vi "Show table.vi"() -> ()   [LabVIEW 2015]
uses:
  <vilib>/addons/database/_DB Variant To Data/Database Variant To Data.xnode
  <vilib>/addons/database/Connection.llb/Conn Execute.vi
  <vilib>/addons/database/Connection.llb/DB Tools Open Connec (Path).vi
  <vilib>/addons/database/Recordset.llb/Rec Destroy - Connection.vi
  <vilib>/addons/database/Recordset.llb/Rec Fetch Recordset Data (R).vi
  <vilib>/addons/database/NI_Database_API.lvlib
panel:
  out "Array":string[][](array[string])
  in  "connection information":path
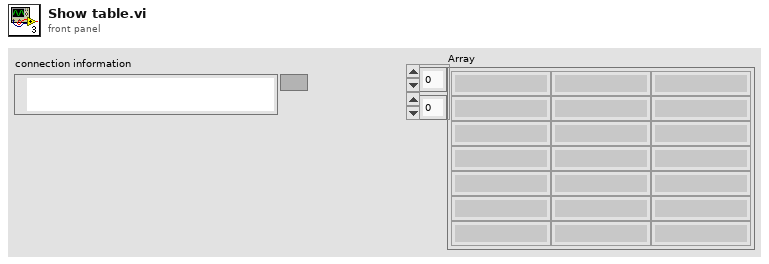
[diagram p1: front panel]
types:
  T1 = typedef "NI_Database_API.lvlib/Conn ObjectReference.ctl" = refnum<k1>
  T2 = typedef "NI_Database_API.lvlib/Rec ObjectReference.ctl" = refnum<k1>
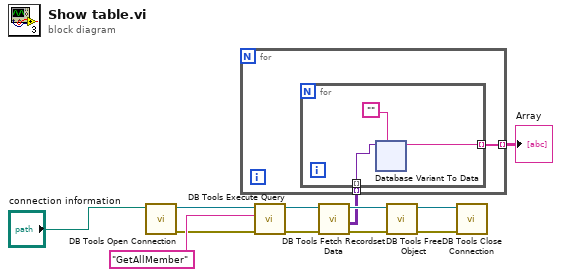
[diagram p0: block diagram]
diagram:
  n1 = call-poly <vilib>:"DB Tools Open Connection.vi"("connection information"="connection information") -> ("error out"=w7:errorcluster, "connection reference"=w8:T1)  [unwired: 7 in]
  n2 = call-poly <vilib>:"DB Tools Execute Query.vi"("error in (no error)"=w7, "SQL query"="GetAllMember", "connection reference"=w8) -> ("error out"=w4:errorcluster, "recordset reference"=w6:T2)  [unwired: 5 in]
  n3 = call-poly <vilib>:"DB Tools Fetch Recordset Data.vi"("error in (no error)"=w4, "recordset reference"=w6) -> ("error out"=w3:errorcluster, "recordset data"=w2:variant[][], "recordset reference out"=w5:T2)  [unwired: 3 in]
  n4 = for {
    tunnel: [w14] -> w1 mode=indexing
    tunnel: w2 -> [w13] mode=indexing
    n5 = for {
      tunnel: [w17] -> w14 mode=indexing
      tunnel: w13 -> [w16] mode=indexing
      n6 = xnode "Database Variant To Data"("database variant"=w16, "type"="") -> ("data"=w17:string)  [unwired: 1 in, 1 out]
    }
  }
  "Array" <- w1
  n7 = call-poly <vilib>:"DB Tools Free Object.vi"("error in (no error)"=w3, "recordset reference"=w5) -> ("error out"=w12:errorcluster, "connection reference"=w11:T1)  [unwired: 8 in]
  n8 = call <vilib>:"DB Tools Close Connection.vi"("error in (no error)"=w12, "connection reference"=w11) -> ()  [unwired: 5 in, 1 out]
